vi "fir_reload_test1.vi"() -> ()   [LabVIEW 2013]
uses:
  <vilib>/Analysis/NI_AALBase.lvlib
panel:
  in  "new coeffs":bool
  out "Array":bool[](array[boolean])
  out "Max Generated":dbl
  out "Simulated":dbl[][](graph)
  in  "stop":bool
  out "Filtered":dbl(graph)
  out "Max":fxp<+/-,16,16>
  out "# of Iterations":i32
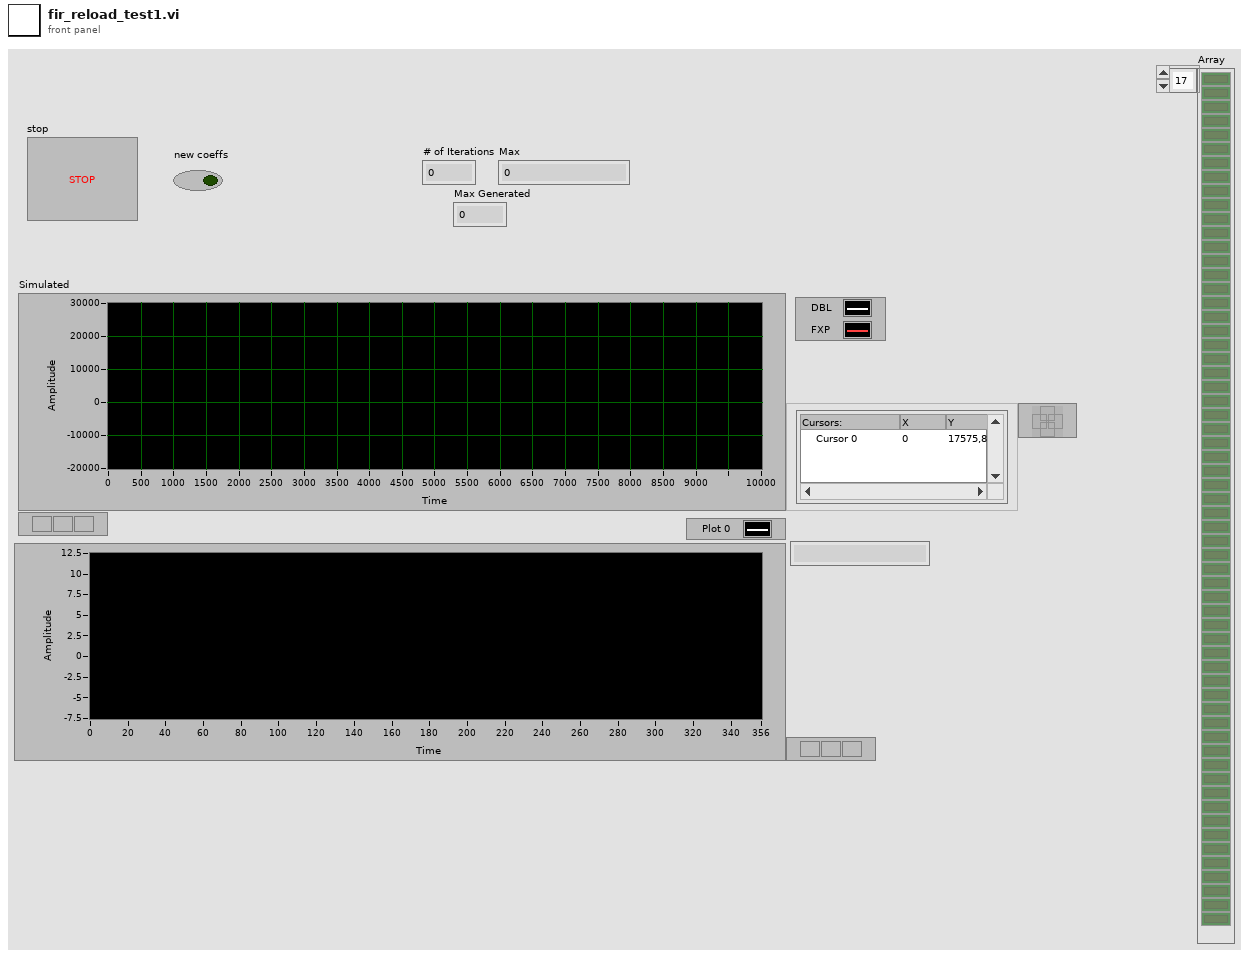
[diagram p1: front panel]
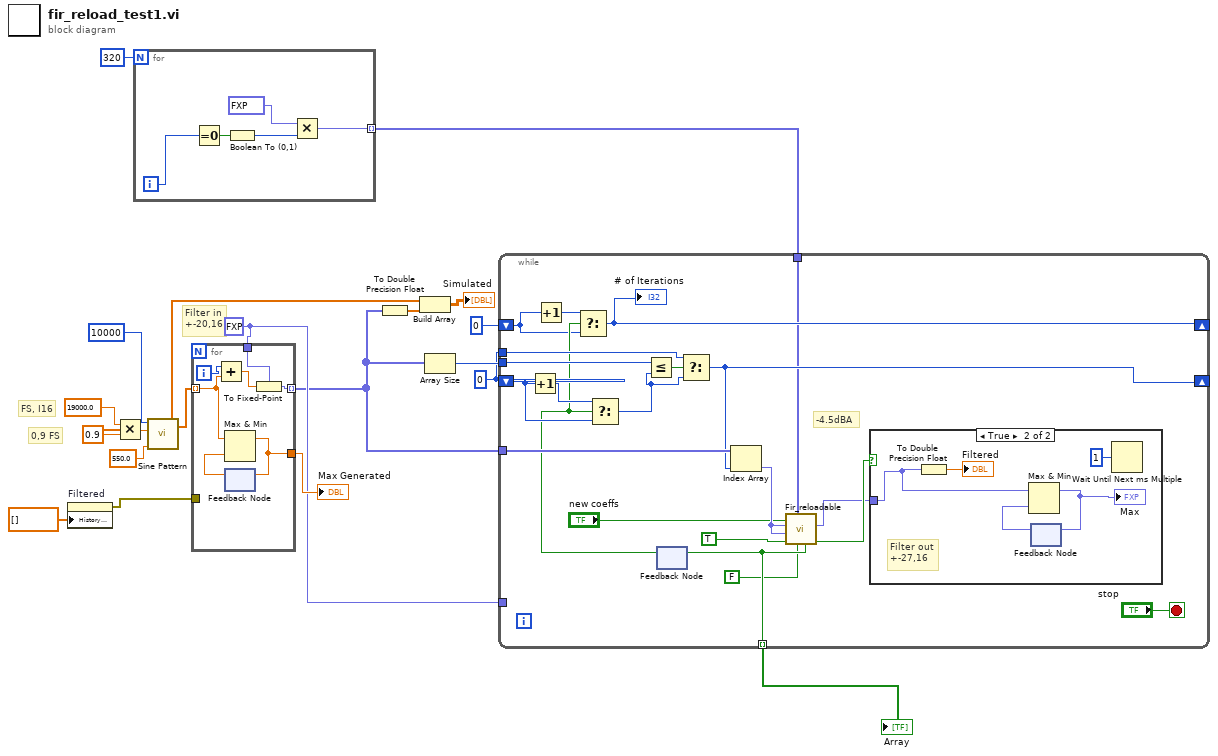
[diagram p0: block diagram]
diagram:
  w6 = fxp<+/-,25,19> 0.0 ("fixed-point type")
  w14 = 0 ("samples")
  # "Filter in\n+-20,16"
  # "FS, I16"
  # "0,9 FS"
  n1 = property on="Filtered" class="WFChart (strict)"("History Data"=dbl[] []) -> (error out=w8:errorcluster)  [unwired: 2 in, 1 out]
  n2 = Multiply(x=19000.0 ("amplitude"), y=0.9) -> (x*y=w16:dbl)
  n3 = for {
    N: 320 -> [_]
    tunnel: [w20] -> w1 mode=indexing
    i -> [w24]
    n4 = Equal To 0?(x=w24) -> (x = 0?=w23:bool)
    n5 = Boolean To (0,1)(Boolean=w23) -> (0, 1=w21:i16)
    n6 = Multiply(x=fxp<+,11,15> 30000.0 ("s_axis_reload_tdata 2"), y=w21) -> (x*y=w20:fxp<+/-,27,31>)
  }
  n7 = call <vilib>:"Sine Pattern.vi"("cycles"=550.0, "amplitude"=w16, "samples"=10000) -> ("Sinusoidal Pattern"=w12:dbl[])  [unwired: 1 in, 1 out]
  n8 = for {
    tunnel: w12 -> [w27] mode=indexing
    tunnel: [w31] -> w4 mode=indexing
    tunnel: w6 -> [w30]
    tunnel: [w28] -> w9
    tunnel: w8 -> [_]
    i -> [w26]
    n9 = Add(x=w26, y=w27) -> (x+y=w25:dbl)
    n10 = feedback #1() -> (w29:dbl)  [unwired: 1 in]
    n11 = Max & Min(x=w27, y=w29) -> (max(x,y)=w28:dbl)  [unwired: 1 out]
    n12 = feedback-in #1(w28) -> ()
    n13 = To Fixed-Point(fixed-point type=w30, number=w25) -> (fixed-point=w31:fxp<+/-,25,19>)
  }
  "Max Generated" <- w9
  n14 = To Double Precision Float(number=w4) -> (double precision float=w13:dbl[])
  n15 = Build Array(w12, w13) -> (→"Simulated":dbl[][])
  n16 = Array Size(array=w4) -> (size(s)=w15:i32)
  n17 = while {
    tunnel: w4 -> [w50]
    shift-right: [w49] -> _
    shift-left: w14 -> [w42]
    tunnel: w15 -> [w48]
    tunnel: w14 -> [w51]
    tunnel: w6 -> [_]
    shift-right: [w38] -> _
    shift-left: 0 ("samples") -> [w37]
    tunnel: [w36] -> w3 mode=indexing
    tunnel: w1 -> [w32]
    stop <- "stop" stop-if-true
    # "-4.5dBA"
    n18 = Increment(x=w42) -> (x+1=w43:i32)
    n19 = Increment(x=w37) -> (x+1=w39:i32)
    n20 = feedback #2() -> (w40:bool)  [unwired: 1 in]
    n21 = Select(t=w39, s=w40, f=w37) -> (s? t:f=w38:i32)
    "# of Iterations" <- w38
    n22 = Select(t=w43, s=w40, f=w42) -> (s? t:f=w41:i32)
    n23 = Less Or Equal?(x=w48, y=w41) -> (x <= y?=w47:bool)
    n24 = Select(t=w51, s=w47, f=w41) -> (s? t:f=w49:i32)
    n25 = Index Array(array=w50, index=w49) -> (element=w46:fxp<+/-,25,19>)
    n26 = call "Fir_reloadable.vi"("reset"=FALSE, "Coeffs"=w32, "valid in"=TRUE, "Q in"=w46, "I in"=w46, "new coeffs"="new coeffs") -> ("valid out"=w45:bool, "I out"=w34:fxp<+/-,16,16>, "ready for input"=w36:bool)  [unwired: 2 in, 1 out]
    n27 = feedback-in #2(w36) -> ()
    n28 = case shown="True" w45 {
      tunnel: w34 -> [_ w53]
      frame False {
      }
      frame True {
        # "Filter out\n+-27,16"
        n29 = To Double Precision Float(number=w53) -> (double precision float=→"Filtered":dbl)
        n30 = feedback #3() -> (w56:fxp<+/-,16,16>)  [unwired: 1 in]
        n31 = Max & Min(x=w53, y=w56) -> (max(x,y)=w55:fxp<+/-,16,16>)  [unwired: 1 out]
        "Max" <- w55
        n32 = feedback-in #3(w55) -> ()
        n33 = Wait Until Next ms Multiple(millisecond multiple=u32 1) -> ()  [unwired: 1 out]
      }
    }
  }
  "Array" <- w3
